vi "TestCSSProperties.vi"(8 "error in (no error)":errorcluster) -> (0 "error out":errorcluster)   [LabVIEW 2019]
uses:
  CSSProperties/CSSProperties.lvclass
  <vilib>/addons/_JKI Toolkits/Caraya/classes/Assert/Assert True.vi
  <vilib>/addons/_JKI Toolkits/Caraya/classes/Assert/Assert False.vi
  <vilib>/addons/_JKI Toolkits/Caraya/classes/Assert/Assert Equal Value_Variant.vi
  <vilib>/addons/_JKI Toolkits/Caraya/classes/Assert/Assert Error.vi
  <vilib>/addons/_JKI Toolkits/Caraya/classes/Test/Test.lvclass
  <vilib>/addons/_JKI Toolkits/Caraya/classes/Assert/Assert.lvclass
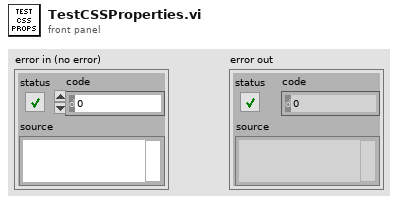
[diagram p1: front panel]
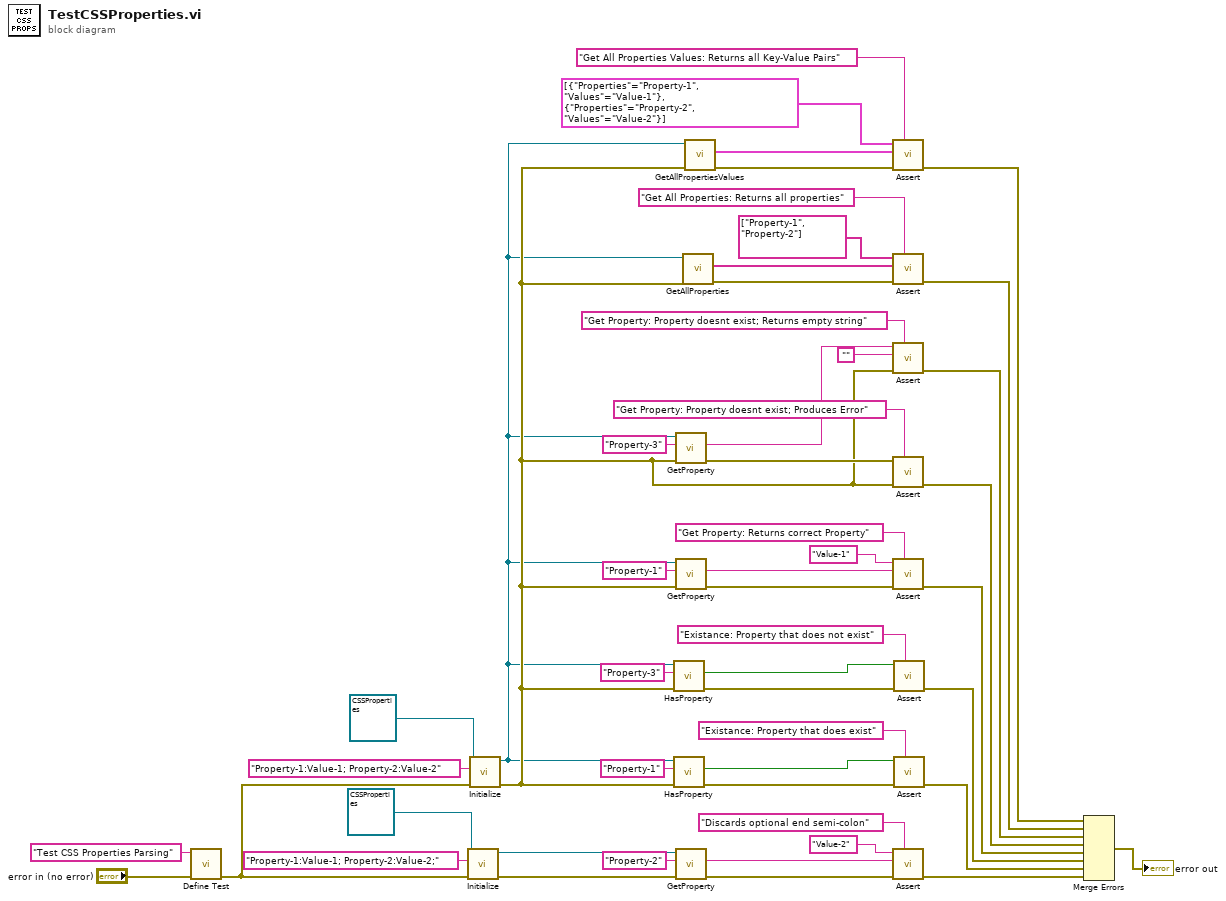
[diagram p0: block diagram]
diagram:
  n1 = call <vilib>:"Define Test.vi"("error in (no error)"="error in (no error)", "Label (VI Title)"="Test CSS Properties Parsing") -> ("error out"=w9:errorcluster)  [unwired: 8 in, 1 out]
  n2 = call "Initialize.vi"("error in (no error)"=w9, "Properties String"="Property-1:Value-1; Property-2:Value-2;", "CSSProperties in"=refnum<class "CSSProperties.lvclass"> refnum) -> ("error out"=w3:errorcluster, "CSSProperties out"=w1:refnum<class "CSSProperties.lvclass">)  [unwired: 7 in]
  n3 = call "Initialize.vi"("error in (no error)"=w9, "Properties String"="Property-1:Value-1; Property-2:Value-2", "CSSProperties in"=refnum<class "CSSProperties.lvclass"> refnum) -> ("error out"=w20:errorcluster, "CSSProperties out"=w19:refnum<class "CSSProperties.lvclass">)  [unwired: 7 in]
  n4 = call "HasProperty.vi"("error in (no error)"=w20, "Property"="Property-3", "CSSProperties in"=w19) -> ("error out"=w40:errorcluster, "Exists?"=w42:bool)  [unwired: 6 in, 1 out]
  n5 = call "HasProperty.vi"("error in (no error)"=w20, "Property"="Property-1", "CSSProperties in"=w19) -> ("error out"=w47:errorcluster, "Exists?"=w45:bool)  [unwired: 6 in, 1 out]
  n6 = call "GetProperty.vi"("error in (no error)"=w20, "Property"="Property-3", "CSSProperties in"=w19) -> ("error out"=w32:errorcluster, "Value"=w31:string)  [unwired: 6 in, 1 out]
  n7 = call "GetProperty.vi"("error in (no error)"=w20, "Property"="Property-1", "CSSProperties in"=w19) -> ("error out"=w39:errorcluster, "Value"=w38:string)  [unwired: 6 in, 1 out]
  n8 = call "GetProperty.vi"("error in (no error)"=w3, "Property"="Property-2", "CSSProperties in"=w1) -> ("error out"=w4:errorcluster, "Value"=w5:string)  [unwired: 6 in, 1 out]
  n9 = call "GetAllProperties.vi"("error in (no error)"=w20, "CSSProperties in"=w19) -> ("error out"=w27:errorcluster, "Properties"=w28:string[])  [unwired: 7 in, 1 out]
  n10 = call "GetAllPropertiesValues.vi"("error in (no error)"=w20, "CSSProperties in"=w19) -> ("error out"=w23:errorcluster, "KVPs"=w22:cluster{"Properties":string, "Values":string}[])  [unwired: 7 in, 1 out]
  n11 = call-poly <vilib>:"Assert.vi"("Label"="Get All Properties Values: Returns all Key-Value Pairs", "error in (no error)"=w23, "Y"=w22, "X"=cluster{"Properties":string, "Values":string}[] [{"Properties"="Property-1", "Values"="Value-1"}, {"Properties"="Property-2", "Values"="Value-2"}] ("KVPs")) -> ("error out"=w13:errorcluster)  [unwired: 6 in, 1 out]
  n12 = call-poly <vilib>:"Assert.vi"("Label"="Get All Properties: Returns all properties", "error in (no error)"=w27, "Y"=w28, "X"=string[] ["Property-1", "Property-2"] ("Properties")) -> ("error out"=w14:errorcluster)  [unwired: 6 in, 1 out]
  n13 = call-poly <vilib>:"Assert.vi"("Label"="Get Property: Property doesnt exist; Returns empty string", "error in (no error)"=w20, "Y"="", "X"=w31) -> ("error out"=w15:errorcluster)  [unwired: 6 in, 1 out]
  n14 = call-poly <vilib>:"Assert.vi"("Label"="Get Property: Property doesnt exist; Produces Error", "error in (no error)"=w20, "Error?"=w32) -> ("error out"=w16:errorcluster)  [unwired: 7 in, 1 out]
  n15 = call-poly <vilib>:"Assert.vi"("Label"="Get Property: Returns correct Property", "error in (no error)"=w39, "Y"=w38, "X"="Value-1") -> ("error out"=w17:errorcluster)  [unwired: 6 in, 1 out]
  n16 = call-poly <vilib>:"Assert.vi"("Label"="Discards optional end semi-colon", "error in (no error)"=w4, "Y"=w5, "X"="Value-2") -> ("error out"=w2:errorcluster)  [unwired: 6 in, 1 out]
  n17 = call-poly <vilib>:"Assert.vi"("Label"="Existance: Property that does not exist", "error in (no error)"=w40, "False?"=w42) -> ("error out"=w18:errorcluster)  [unwired: 7 in, 1 out]
  n18 = call-poly <vilib>:"Assert.vi"("Label"="Existance: Property that does exist", "error in (no error)"=w47, "True?"=w45) -> ("error out"=w10:errorcluster)  [unwired: 7 in, 1 out]
  n19 = Merge Errors(w13, w14, w15, w16, w17, w18, w10, w2) -> (→"error out":errorcluster)
